vi "WinUCHAR.vi"() -> ()   [LabVIEW 2023]
doc: "This function reverses the input string and places it in output.\n\nFor information on the data types used for the DLL function, right-click on the Call Library Function node and choose Configure."
uses:
  CLF_Example.dll
panel:
  out "output":string
  in  "input":string="abcd"
  # "Please use alphanumeric characters to get proper results."
  # "See the block diagram for more information."
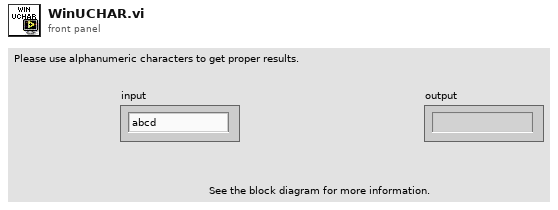
[diagram p1: front panel]
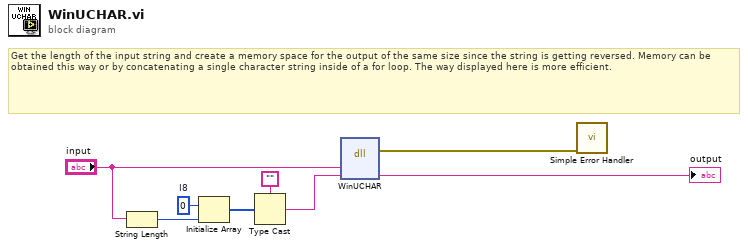
[diagram p0: block diagram]
diagram:
  w7 = u8 0  # I8
  # "Get the length of the input string and create a memory space for the output of the same size since the string is getting reversed. Memory can be obtained this way or by concatenating a single character string inside of a for loop. The way displayed here is more efficient."
  n1 = String Length(string="input") -> (length=w6:i32)
  n2 = Initialize Array(w7, w6) -> (w4:u8[])
  n3 = Type Cast(type="", x=w4) -> (*(type *) &x=w2:string)
  n4 = dll-call lib="c:/dev/_r/4/eng/lv-core/lvpostprocessingd/lv_mc_x86_64/dist_i386/examples/Connectivity/Libraries and Executables/DLL Calling VIs/CLF_Example**.*" fn="WinUCHAR"("input"="input", "output"=w2) -> (error out=w1:errorcluster, "output"=→"output":string)  [unwired: 3 in, 3 out]
  n5 = call <vilib>:"Simple Error Handler.vi"("error in (no error)"=w1) -> ()  [unwired: 4 in, 5 out]
